vi "NI VeriStand - Get Stimulus Profile Result.vi"(8 "error in (no error)":errorcluster, 11 "StimulusProfileManager in":T2) -> (0 "error out":errorcluster, 1 "Result File":path, 2 "Result":T1, 3 "StimulusProfileManager out":T2)   [LabVIEW 2020, in "NI_VS Stimulus ExecutionAPI.lvlib"]
doc: "This VI interfaces with the legacy Stimulus Profile Editor workspace tool in NI VeriStand, and is included for compatibility only. National Instruments recommends you use the current Stimulus Profile VIs to create, observe, and control NI VeriStand stimulus profiles and real-time sequences.\n\nReturns the results of the last stimulus profile file that ran on the target, including whether it passed, failed, or received an error."
uses:
  <vilib>/NI VeriStand/Execution/Stimulus/NI_VS Stimulus ExecutionAPI.lvlib
  <vilib>/NI VeriStand/Execution/Stimulus/StimulusAPI.ctl
  NationalInstruments.VeriStand.ClientAPI
  <vilib>/NI VeriStand/Execution/Stimulus/StimulusResult.ctl
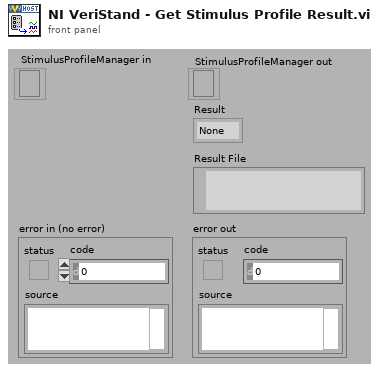
[diagram p1: front panel]
types:
  T1 = typedef "NI_VS Stimulus ExecutionAPI.lvlib/StimulusResult.ctl" = enum16{"None", "Passed", "Failed", "Error"}
  T2 = typedef "NI_VS Stimulus ExecutionAPI.lvlib/StimulusAPI.ctl" = refnum<k24>
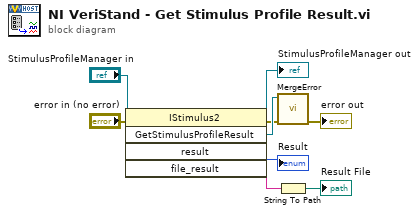
[diagram p0: block diagram]
diagram:
  n1 = invoke class="IStimulus2" method="GetStimulusProfileResult"(reference="StimulusProfileManager in", error in="error in (no error)") -> (reference out=→"StimulusProfileManager out":T2, error out=w6:errorcluster, "GetStimulusProfileResult"=w7:refnum<k24>, "result"=→"Result":u8, "file_result"=w4:string)  [unwired: 3 in]
  n2 = call <vilib>:"MergeError.vi"("error in (no error)"=w6, "Error"=w7) -> ("error out"=→"error out":errorcluster)  [unwired: 9 out]
  n3 = String To Path(string=w4) -> (path=→"Result File":path)
